vi "Test shm get Response set Auth List LV.vi"(8 "error in (no error)":errorcluster, 11 "ackcmd_Ctl":T1) -> (0 "error out":errorcluster, 2 "function return":i32, 3 "ackcmd_Ctl out":T1)   [LabVIEW 2018, in "SALLV_Test.lvlib"]
doc: "int Test_shm_getResponse_setAuthListLV(Test_ackcmdLV *ackcmd_Ctl);"
uses:
  SALLV_Test.lvlib
  SALLV_Test.so
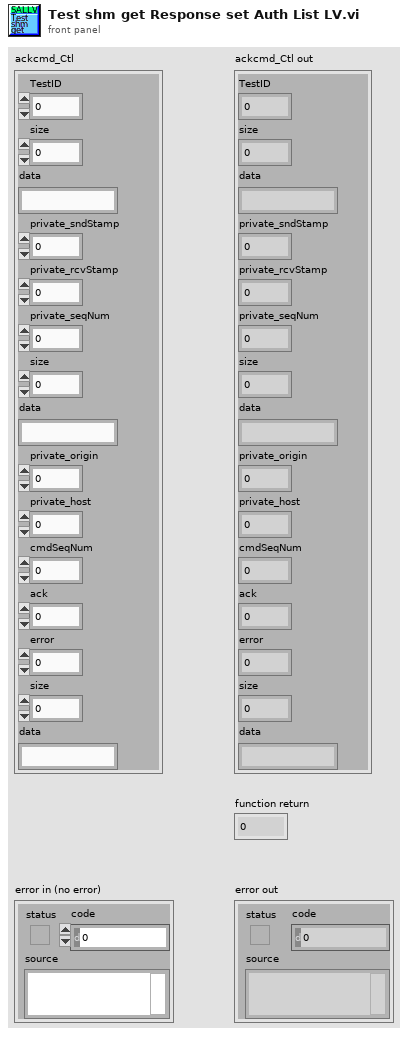
[diagram p1: front panel]
types:
  T1 = cluster{"TestID":i32, "size":i32, "data":string, "private_sndStamp":dbl, "private_rcvStamp":dbl, "private_seqNum":i32, "size":i32, "data":string, "private_origin":i32, "private_host":i32, "cmdSeqNum":i32, "ack":i32, "error":i32, "size":i32, "data":string}
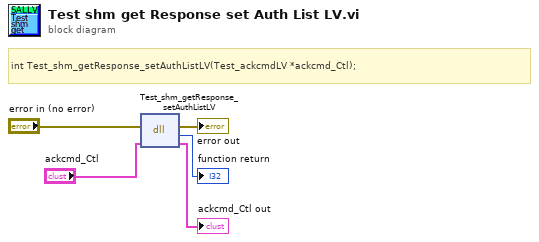
[diagram p0: block diagram]
diagram:
  # "int Test_shm_getResponse_setAuthListLV(Test_ackcmdLV *ackcmd_Ctl);"
  n1 = dll-call lib="home/ttsai/Documents/salTestLabViewApi/SALLV_Test/SALLV_Test.*" fn="Test_shm_getResponse_setAuthListLV"(error in="error in (no error)", "ackcmd_Ctl"="ackcmd_Ctl") -> (error out=→"error out":errorcluster, →"function return":i32, "ackcmd_Ctl"=→"ackcmd_Ctl out":T1)  [unwired: 2 in, 1 out]
